vi "Horizontal Mirror.vi"(7 "N":i32, 10 "Mirror Position":i32, 11 "Rocks":cluster{i32, i32}[](array[cluster])) -> (2 "Mirror?":bool, 3 "Rows":u64)   [LabVIEW 2023, in "d13.lvlib"]
uses:
  d13.lvlib
  a4cb4a31-daad-49c2-a719-03c442b6ebeb.vi
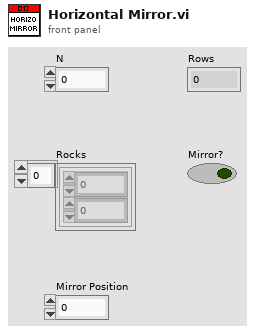
[diagram p1: front panel]
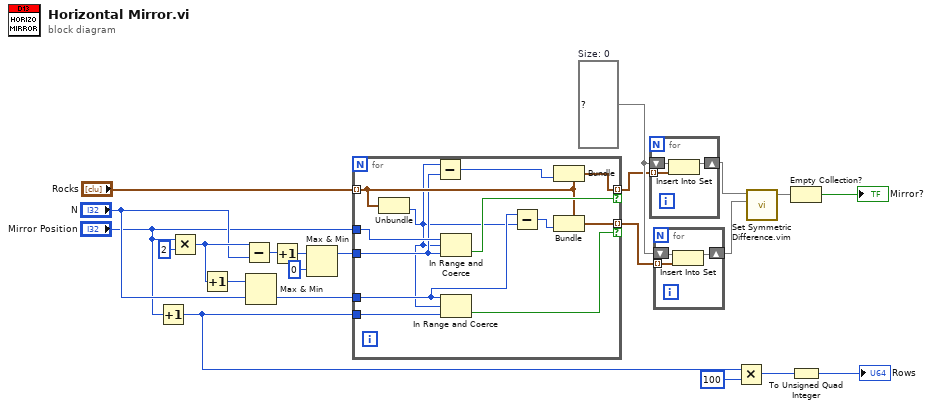
[diagram p0: block diagram]
diagram:
  w22 = set{cluster{"offset of match":i32, i32}} {}  # Size: 0
  n1 = Increment(x="Mirror Position") -> (x+1=w21:i32)
  n2 = Multiply(x="Mirror Position", y=2) -> (x*y=w15:i32)
  n3 = Increment(x=w15) -> (x+1=w18:i32)
  n4 = Subtract(x=w15, y="N") -> (x-y=w10:i32)
  n5 = Max & Min(x=w18, y="N") -> (min(x,y)=w16:i32)  [unwired: 1 out]
  n6 = Increment(x=w10) -> (x+1=w11:i32)
  n7 = Max & Min(x=w11, y=0) -> (max(x,y)=w12:i32)  [unwired: 1 out]
  n8 = for {
    tunnel: "Rocks" -> [w31] mode=indexing
    tunnel: [w30] -> w7 mode=indexing if=w32
    tunnel: [w34] -> w17 mode=indexing if=w33
    tunnel: w12 -> [w28]
    tunnel: "Mirror Position" -> [w29]
    tunnel: w21 -> [w27]
    tunnel: w16 -> [w26]
    n9 = Unbundle(w31) -> (w23:i32)  [unwired: 1 out]
    n10 = Subtract(x=w23, y=w28) -> (x-y=w25:i32)
    n11 = In Range and Coerce(upper limit=w29, x=w23, lower limit=w28) -> (In Range?=w32:bool)  [unwired: 1 out]
    n12 = In Range and Coerce(upper limit=w26, x=w23, lower limit=w27) -> (In Range?=w33:bool)  [unwired: 1 out]
    n13 = Subtract(x=w26, y=w23) -> (x-y=w24:i32)
    n14 = Bundle(cluster=w31, w25) -> (w30:cluster{i32, i32})  [unwired: 1 in]
    n15 = Bundle(cluster=w31, w24) -> (w34:cluster{i32, i32})  [unwired: 1 in]
  }
  n16 = for {
    tunnel: w7 -> [w36] mode=indexing
    shift-right: [w35] -> w3
    shift-left: w22 -> [w37]
    n17 = Insert Into Set(10:w36, 11:w37) -> (3:w35:set{cluster{"offset of match":i32, i32}})  [unwired: 1 out]
  }
  n18 = for {
    tunnel: w17 -> [w39] mode=indexing
    shift-right: [w38] -> w2
    shift-left: w22 -> [w40]
    n19 = Insert Into Set(10:w39, 11:w40) -> (3:w38:set{cluster{"offset of match":i32, i32}})  [unwired: 1 out]
  }
  n20 = Multiply(x=w21, y=100) -> (x*y=w19:i32)
  n21 = call "Set Symmetric Difference.vim"("set 2"=w2, "set 1"=w3) -> ("symmetric difference"=w4:set{cluster{"offset of match":i32, i32}})  [unwired: 9 in]
  n22 = Empty Collection?(1:w4) -> (0:→"Mirror?":bool)
  n23 = To Unsigned Quad Integer(1:w19) -> (0:→"Rows":u64)
